vi "FileIO-Check Overwrite.vi"(0 "path":path, 11 "error in (no error)":errorcluster) -> (4 "path thru":path, 8 "Conitnue?":bool, 15 "error out":errorcluster)   [LabVIEW 2020]
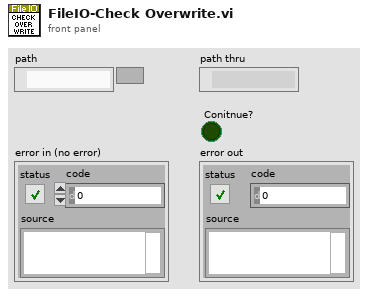
[diagram p1: front panel]
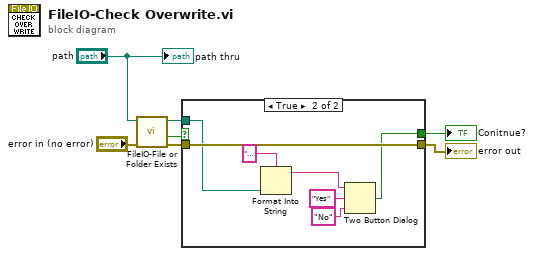
[diagram p0: block diagram]
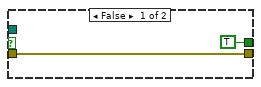
[diagram p2: hidden frame]
diagram:
  n1 = call "FileIO-File or Folder Exists.vi"("error in (no error)"="error in (no error)", "path"="path") -> ("error out"=w6:errorcluster, "Exists?"=w3:bool, "dup path"=w1:path)  [unwired: 6 in, 1 out]
  n2 = case shown="True" w3 {
    tunnel: [w9 w16] -> w5
    tunnel: w6 -> [w9 w16]
    tunnel: [TRUE w13] -> w7
    tunnel: w1 -> [_ w12]
    frame False {
    }
    frame True {
      n3 = Format Into String(format string="File exists: \n'%s'\n\nOverwrite file?", w12) -> (resulting string=w11:string)  [unwired: 2 in, 1 out]
      n4 = Two Button Dialog(message=w11, 1:"No" ("F button name (\"Cancel\")"), 2:"Yes" ("T button name (\"OK\")")) -> (T button?=w13:bool)
    }
  }
  "Conitnue?" <- w7
  "error out" <- w5
  "path thru" <- "path"
